vi "Read Characters From File.vi"(5 "convert eol? (no:F)":bool, 8 "error in":errorcluster, 9 "start of read offset (chars.:0)":i32, 10 "number of characters (all:-1)":i32=-1, 11 "file path (dialog if empty)":path) -> (0 "error out":errorcluster, 2 "EOF?":bool, 3 "new file path (NotAPath if cancelled)":path, 4 "mark after read (chars.)":i32, 6 "character string":string)   [LabVIEW 2011]
doc: "LabVIEW no longer supports this VI. Use the Read Text function instead. Reads a specified number of characters from a byte stream file beginning at a specified character offset. The VI opens the file before reading from it and closes it afterwards."
uses:
  <vilib>/Utility/error.llb/DialogType.ctl
panel:
  in  "prompt":string="Choose file to read."
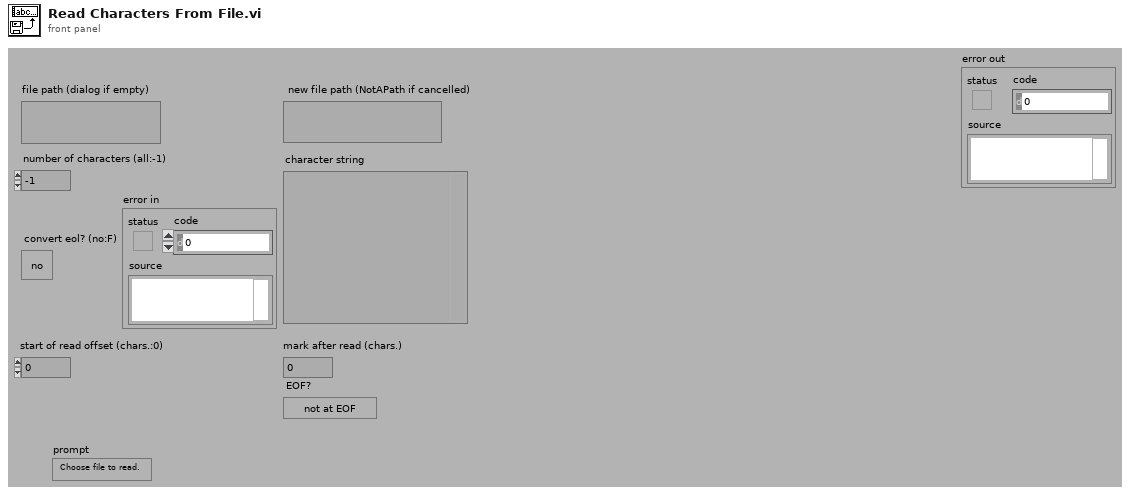
[diagram p1: front panel]
types:
  T1 = typedef "DialogType.ctl" = u16
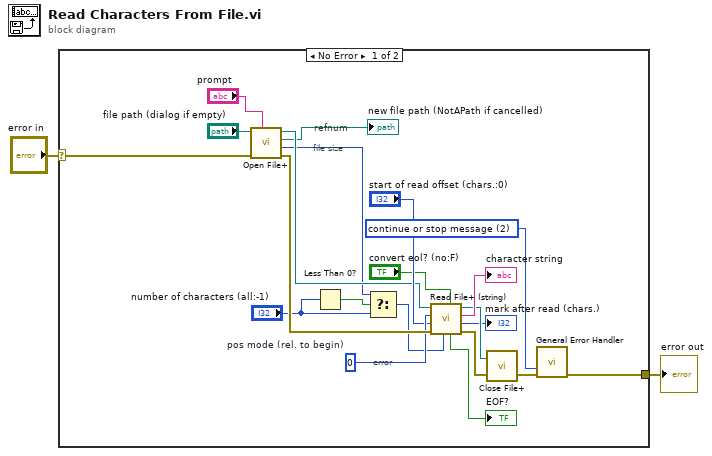
[diagram p0: block diagram]
diagram:
  n1 = case shown="No Error" "error in" {
    selector: "error in" -> [w4 w24]
    tunnel: [w3 w24] -> w1
    frame No Error {
      w5 = T1 2 items=["no dialog", "OK message", "continue or stop message", "OK message + warnings", "continue/stop + warnings"] ("type of dialog (OK msg:1)")
      w20 = i16 0  # pos mode (rel. to begin)
      # "file size"
      # "error"
      # "refnum"
      n2 = call <vilib>:"Open File+.vi"("prompt"="prompt", "error in (not an error)"=w4, "file path (\" \")"="file path (dialog if empty)") -> ("error out"=w22:errorcluster, "file size (bytes)"=w10:i32, "file path"=→"new file path (NotAPath if cancelled)":path, "refnum"=w13:refnum<file>)  [unwired: 5 in]
      n3 = Less Than 0?(x="number of characters (all:-1)") -> (x < 0?=w11:bool)
      n4 = Select(t=w10, s=w11, f="number of characters (all:-1)") -> (s? t:f=w8:i32)
      n5 = call <vilib>:"Read File+ (string).vi"("convert eol? (no:F)"="convert eol? (no:F)", "count"=w8, "error in (no error)"=w22, "pos offset (bytes:0)"="start of read offset (chars.:0)", "pos mode (rel. to current:2)"=w20, "refnum"=w13) -> ("error out"=w18:errorcluster, "mark after read (bytes)"=→"mark after read (chars.)":i32, "string"=→"character string":string, "dup refnum"=w17:refnum<file>, "EOF?"=→"EOF?":bool)  [unwired: 1 in]
      n6 = call <vilib>:"Close File+.vi"("error in (no error)"=w18, "refnum"=w17) -> ("error out"=w15:errorcluster)  [unwired: 3 in, 2 out]
      n7 = call <vilib>:"General Error Handler.vi"("type of dialog (OK msg:1)"=w5, "error in (no error)"=w15) -> ("error out"=w3:errorcluster)  [unwired: 9 in, 4 out]
    }
    frame Error {
    }
  }
  "error out" <- w1
